vi "API - Stream - Download ADC and DIO Data.vi"(8 "error in":errorcluster, 11 "DAQiFi Device Properties In":T1) -> (0 "error out":errorcluster, 1 "Digital Inputs":bool[](array[boolean]), 2 "Array of Voltages (V)":dbl[](array[numeric]), 3 "DAQiFi Device Properties Out":T1)   [LabVIEW 2021]
doc: "Download a single data point from an array of ADC channels and digital channels.\nThe index of the voltages array is the channel number of the analog input.\nThe index of the digital inputs array is the channel number of the digital input."
uses:
  TypeDefs/TypeDef - Cluster of DAQiFi Device Properties.ctl
  TypeDefs/Enum - Connection Type.ctl
  TCP - Asynchronous Read of One JSON Message.vi
  USB - Asynchronous Read of One JSON Message.vi
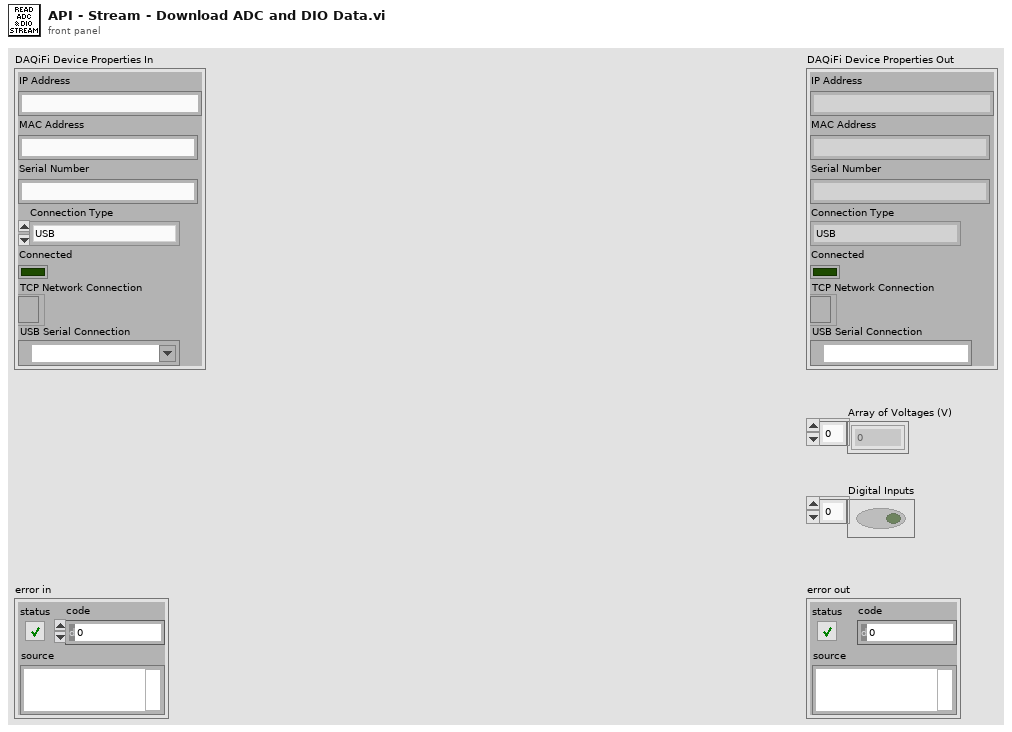
[diagram p1: front panel]
types:
  T1 = typedef "TypeDef - Cluster of DAQiFi Device Properties.ctl" = cluster{"IP Address":string, "MAC Address":string, "Serial Number":string, "Connection Type":T2, "Connected":bool, "TCP Network Connection":refnum<k5>, "USB Serial Connection":refnum<visa-resource-name>}
  T2 = typedef "Enum - Connection Type.ctl" = enum16{"USB", "TCP"}
  T3 = typedef "TypeDef - Cluster Representing Decoded JSON Message.ctl" = cluster{"timestamp":u64, "adc":cluster{"time":i32, "ch":i32, "data":i32}[], "dio":cluster{"time":i32, "mask":i32, "data":u16}[]}
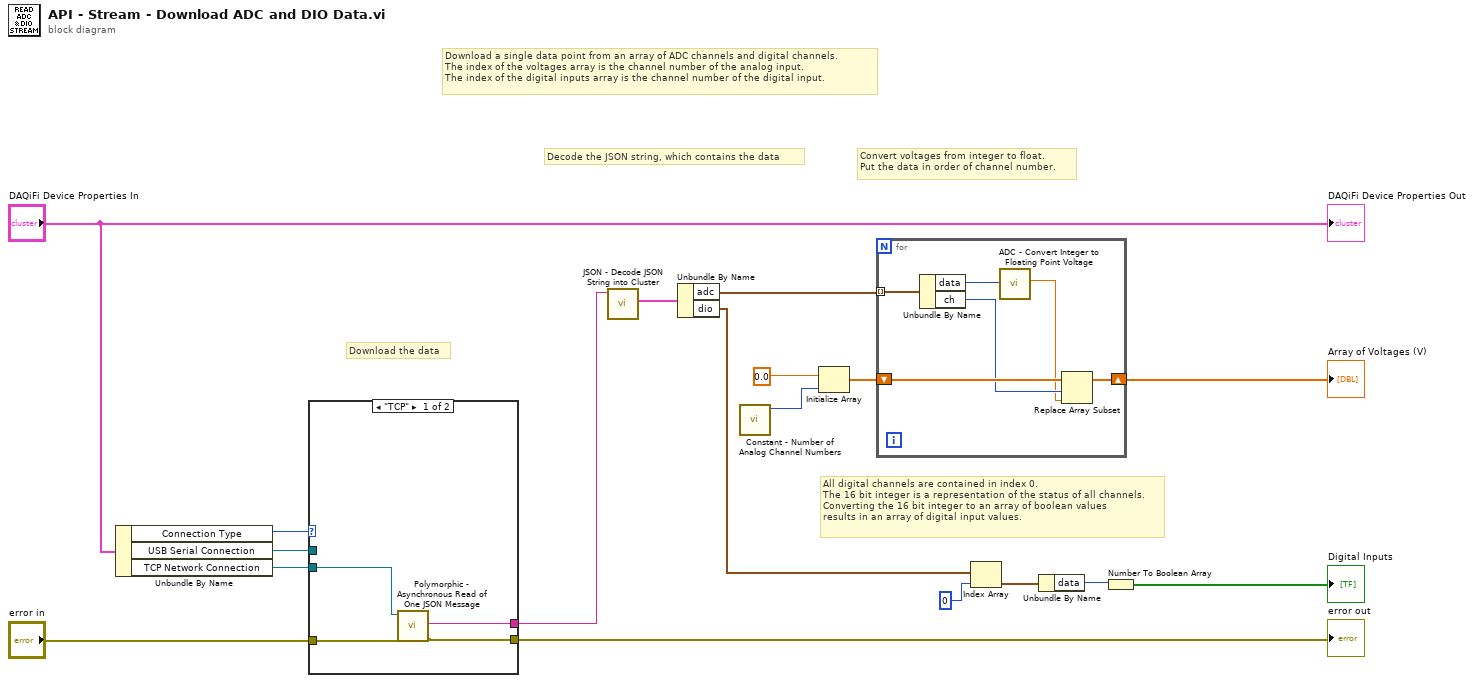
[diagram p0: block diagram]
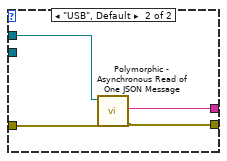
[diagram p2: hidden frame]
diagram:
  # "All digital channels are contained in index 0.\nThe 16 bit integer is a representation of the status of all channels.\nConverting the 16 bit integer to an array of boolean values \nresults in an array of digital input values."
  # "Convert voltages from integer to float.\nPut the data in order of channel number."
  # "Download a single data point from an array of ADC channels and digital channels.\nThe index of the voltages array is the channel number of the analog input.\nThe index of the digital inputs array is the channel number of the digital input."
  # "Decode the JSON string, which contains the data"
  # "Download the data"
  n1 = Unbundle By Name("DAQiFi Device Properties In") -> ("Connection Type"=w3:T2, "USB Serial Connection"=w1:refnum<visa-resource-name>, "TCP Network Connection"=w2:refnum<k5>)
  n2 = case shown="\"TCP\"" w3 {
    tunnel: "error in" -> [w22 w26]
    tunnel: [w21 w25] -> w6
    tunnel: [w20 w24] -> w5
    tunnel: w2 -> [w19 _]
    tunnel: w1 -> [_ w23]
    frame "TCP" {
      n3 = call-poly "Polymorphic - Asynchronous Read of One JSON Message.vi"("error in"=w22, "TCP Network Connection in"=w19) -> ("error out"=w21:errorcluster, "Received JSON Message"=w20:string)  [unwired: 7 in, 1 out]
    }
    frame "USB", Default {
      n4 = call-poly "Polymorphic - Asynchronous Read of One JSON Message.vi"("error in"=w26, "VISA resource name in"=w23) -> ("error out"=w25:errorcluster, "Received JSON Message"=w24:string)  [unwired: 7 in, 1 out]
    }
  }
  "error out" <- w6
  n5 = call "JSON - Decode JSON String into Cluster.vi"("JSON String"=w5) -> ("Data out"=w18:T3)  [unwired: 9 in, 1 out]
  n6 = Unbundle By Name(w18) -> ("adc"=w17:cluster{"time":i32, "ch":i32, "data":i32}[], "dio"=w8:cluster{"time":i32, "mask":i32, "data":u16}[])
  n7 = call "Constant - Number of Analog Channel Numbers.vi"() -> ("Maximum Channel"=w13:i32)  [unwired: 11 in]
  n8 = Initialize Array(0.0, w13) -> (w15:dbl[])
  n9 = for {
    tunnel: w17 -> [w32] mode=indexing
    shift-right: [w27] -> w14
    shift-left: w15 -> [w30]
    n10 = Unbundle By Name(w32) -> ("data"=w31:i32, "ch"=w29:i32)
    n11 = call "ADC - Convert Integer to Floating Point Voltage.vi"("Analog Integer Value In"=w31) -> ("Analog Voltage (V)"=w28:dbl)  [unwired: 10 in]
    n12 = Replace Array Subset(array=w30, new element=w28, index=w29) -> (w27:dbl[])
  }
  "Array of Voltages (V)" <- w14
  n13 = Index Array(array=w8, index=0) -> (element=w11:cluster{"time":i32, "mask":i32, "data":u16})
  n14 = Unbundle By Name(w11) -> ("data"=w10:u16)
  n15 = Number To Boolean Array(number=w10) -> (Boolean array=→"Digital Inputs":bool[])
  "DAQiFi Device Properties Out" <- "DAQiFi Device Properties In"
